vi "ChooseOffensivePlay_v2.vi"(0 "object in":refnum<class "Game.lvclass">, 2 "GameRef":refnum<data-value>, 5 "error in (no error)":errorcluster) -> (14 "object out":refnum<class "Game.lvclass">, 19 "error out":errorcluster)   [LabVIEW 2023, in "Game.lvclass"]
uses:
  Game.lvclass
  Game.lvclass/Game.ctl
  NewSTP/Playbook_v2_class/Playbook_v2.lvclass
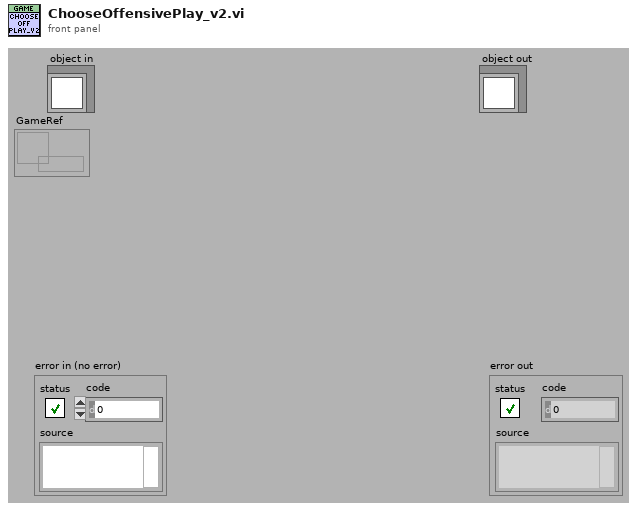
[diagram p1: front panel]
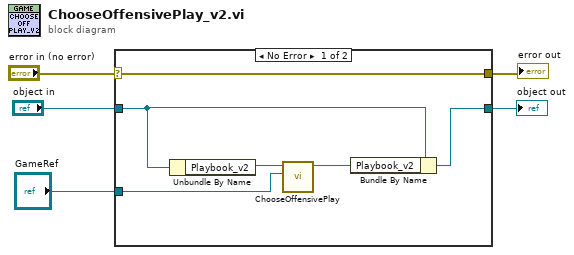
[diagram p0: block diagram]
diagram:
  n1 = case shown="No Error" "error in (no error)" {
    selector: "error in (no error)" -> [w11 w13]
    tunnel: [w11 w13] -> w4
    tunnel: [w9 w12] -> w2
    tunnel: "object in" -> [w7 w12]
    tunnel: "GameRef" -> [w6 _]
    frame No Error {
      n2 = Unbundle By Name(w7) -> ("Playbook_v2"=w10:refnum<class "Playbook_v2.lvclass">)
      n3 = call-dynamic "ChooseOffensivePlay.vi"("GameRef"=w6, "Playbook_v2 in"=w10) -> ("Playbook_v2 out"=w8:refnum<class "Playbook_v2.lvclass">)  [unwired: 8 in, 1 out]
      n4 = Bundle By Name(cluster=w7, "Playbook_v2"=w8) -> (w9:refnum<class "Game.lvclass">)
    }
    frame Error {
    }
  }
  "error out" <- w4
  "object out" <- w2
